vi "Main Panel.vi"() -> ()   [LabVIEW 2014]
panel:
  out "Omar":dbl(slide) scale=0.0..10.0
  out "Mina":dbl(slide) scale=0.0..10.0
  out "Nagy":dbl(slide) scale=0.0..10.0
  out "Shady":dbl(slide) scale=0.0..10.0
  out "Fady":dbl(slide) scale=0.0..10.0
  in  "Stop Button":bool
  # "Destributed Systems\n(Main Panel)"
  # "Client 1"
  # "Client 2"
  # "Client 3"
  # "Client 4"
  # "Client 5"
  # "Exit"
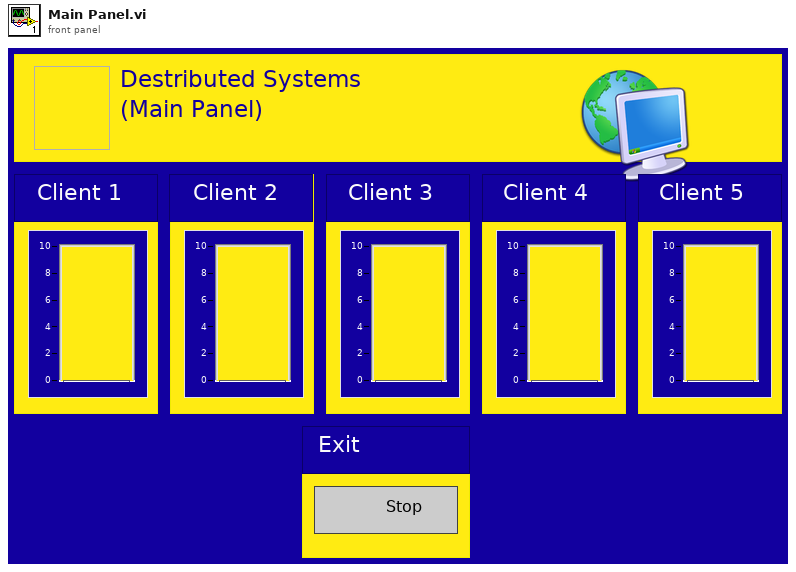
[diagram p1: front panel]
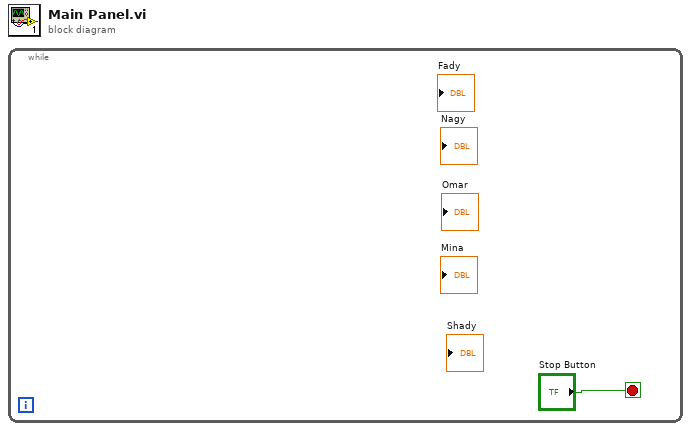
[diagram p0: block diagram]
diagram:
  n1 = while {
    stop <- "Stop Button" stop-if-true
  }
